vi "pause.vi"(8 "error in":errorcluster) -> (0 "error out":errorcluster)   [LabVIEW 2020, in "main.lvlib" / "stopwatch_timer.lvlib"]
uses:
  stopwatch_timer.lvlib
  state.ctl
  library_variable.vi
panel:
  # "Development\ncontrols/indicators useful for development and testing, but which are not outputs of the VI"
  # "Input\nInputs to the VI"
  # "Output\nOutputs of the VI"
  # "Description\n\nBlank VI with error handling case. \n\nSummarize the use of this VI in this space."
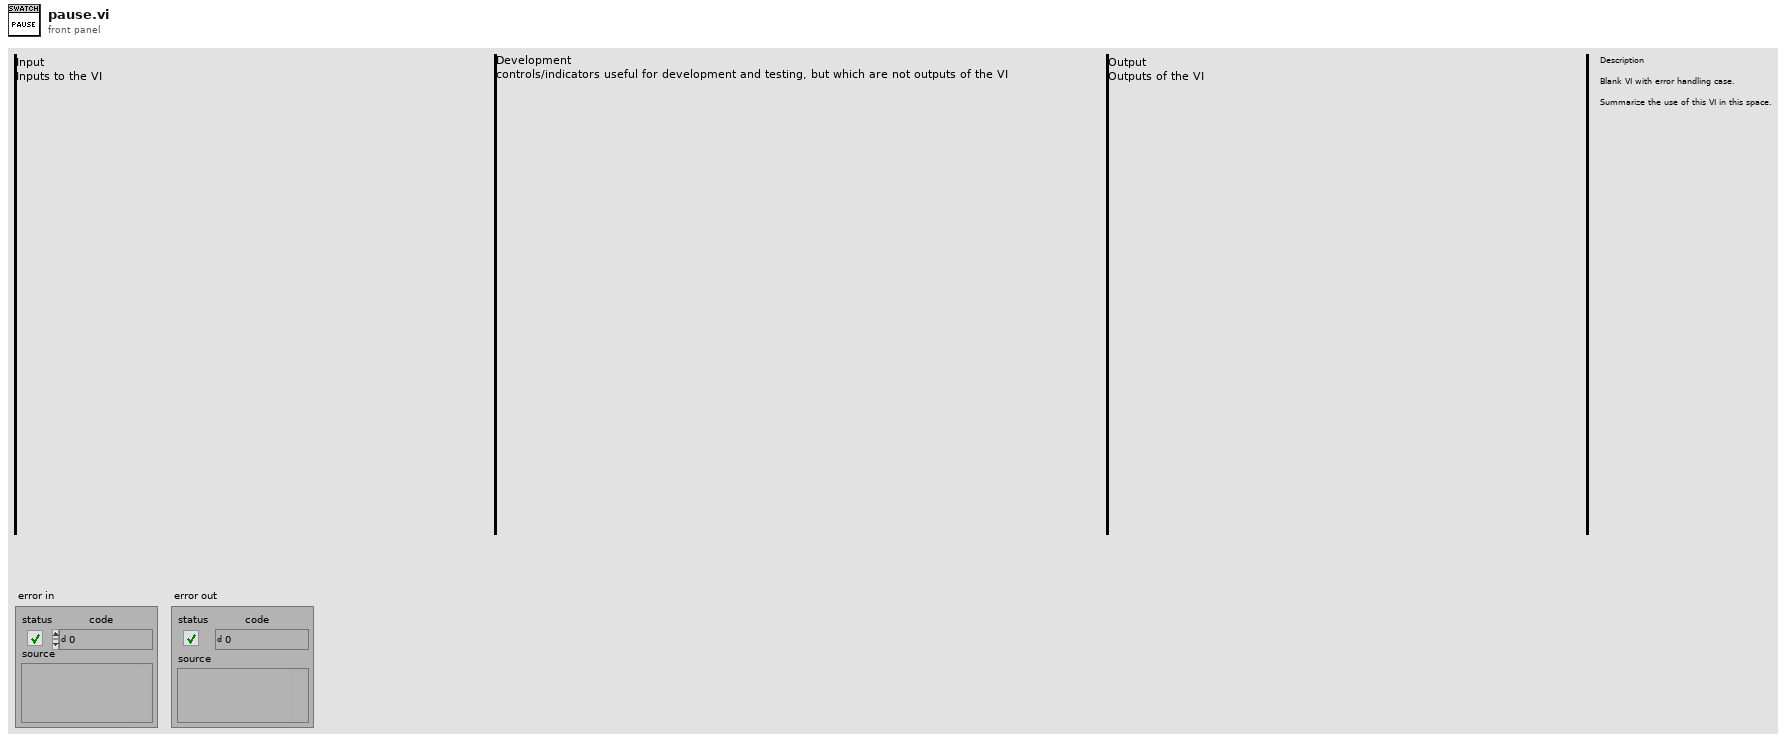
[diagram p1: front panel]
types:
  T1 = typedef "main.lvlib/stopwatch_timer.lvlib/state.ctl" = enum16{"not started", "running", "paused"}
  T2 = typedef "main.lvlib/stopwatch_timer.lvlib/stopwatch data.ctl" = cluster{"state":T1, "started at":timestamp, "last resumed at":timestamp, "last paused at":timestamp, "total time running (seconds)":dbl, "total time paused (seconds)":dbl}
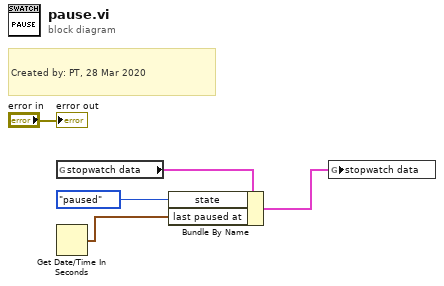
[diagram p0: block diagram]
diagram:
  # "Created by: PT, 28 Mar 2020"
  n1 = global read "library_variable.vi" "stopwatch data"() -> (w3:T2)
  n2 = Get Date/Time In Seconds() -> (seconds since 1Jan1904=w4:timestamp)
  n3 = Bundle By Name(cluster=w3, "state"=state."paused", "last paused at"=w4) -> (w2:T2)
  n4 = global write "library_variable.vi" "stopwatch data"(w2) -> ()
  "error out" <- "error in"
